vi "start scan.vi"(0 "Experiment name":string, 2 "Scan Number":i32, 5 "Scan":T3 {"Scan setup"."Scan Start" format="%#.9p"; "Scan setup"."Scan End" format="%#.9p"; "Scan setup"."Scan Step Size" format="%#.9p"}, 7 "Network":T5, 12 "BG override":bool, 13 "number BG shots DB":i32, 14 "No of BackGround Shots":i32=2) -> (4 "Scan out":T3 {"Scan setup"."Scan Start" format="%#.9p"; "Scan setup"."Scan End" format="%#.9p"; "Scan setup"."Scan Step Size" format="%#.9p"}, 6 "DoScan":bool, 8 "Network out":T5)   [LabVIEW 2018]
uses:
  MCports.ctl
  Scan Tab Enum.ctl
  scan parameters.ctl
  Shared/MySQL/Preset Query Enum.ctl
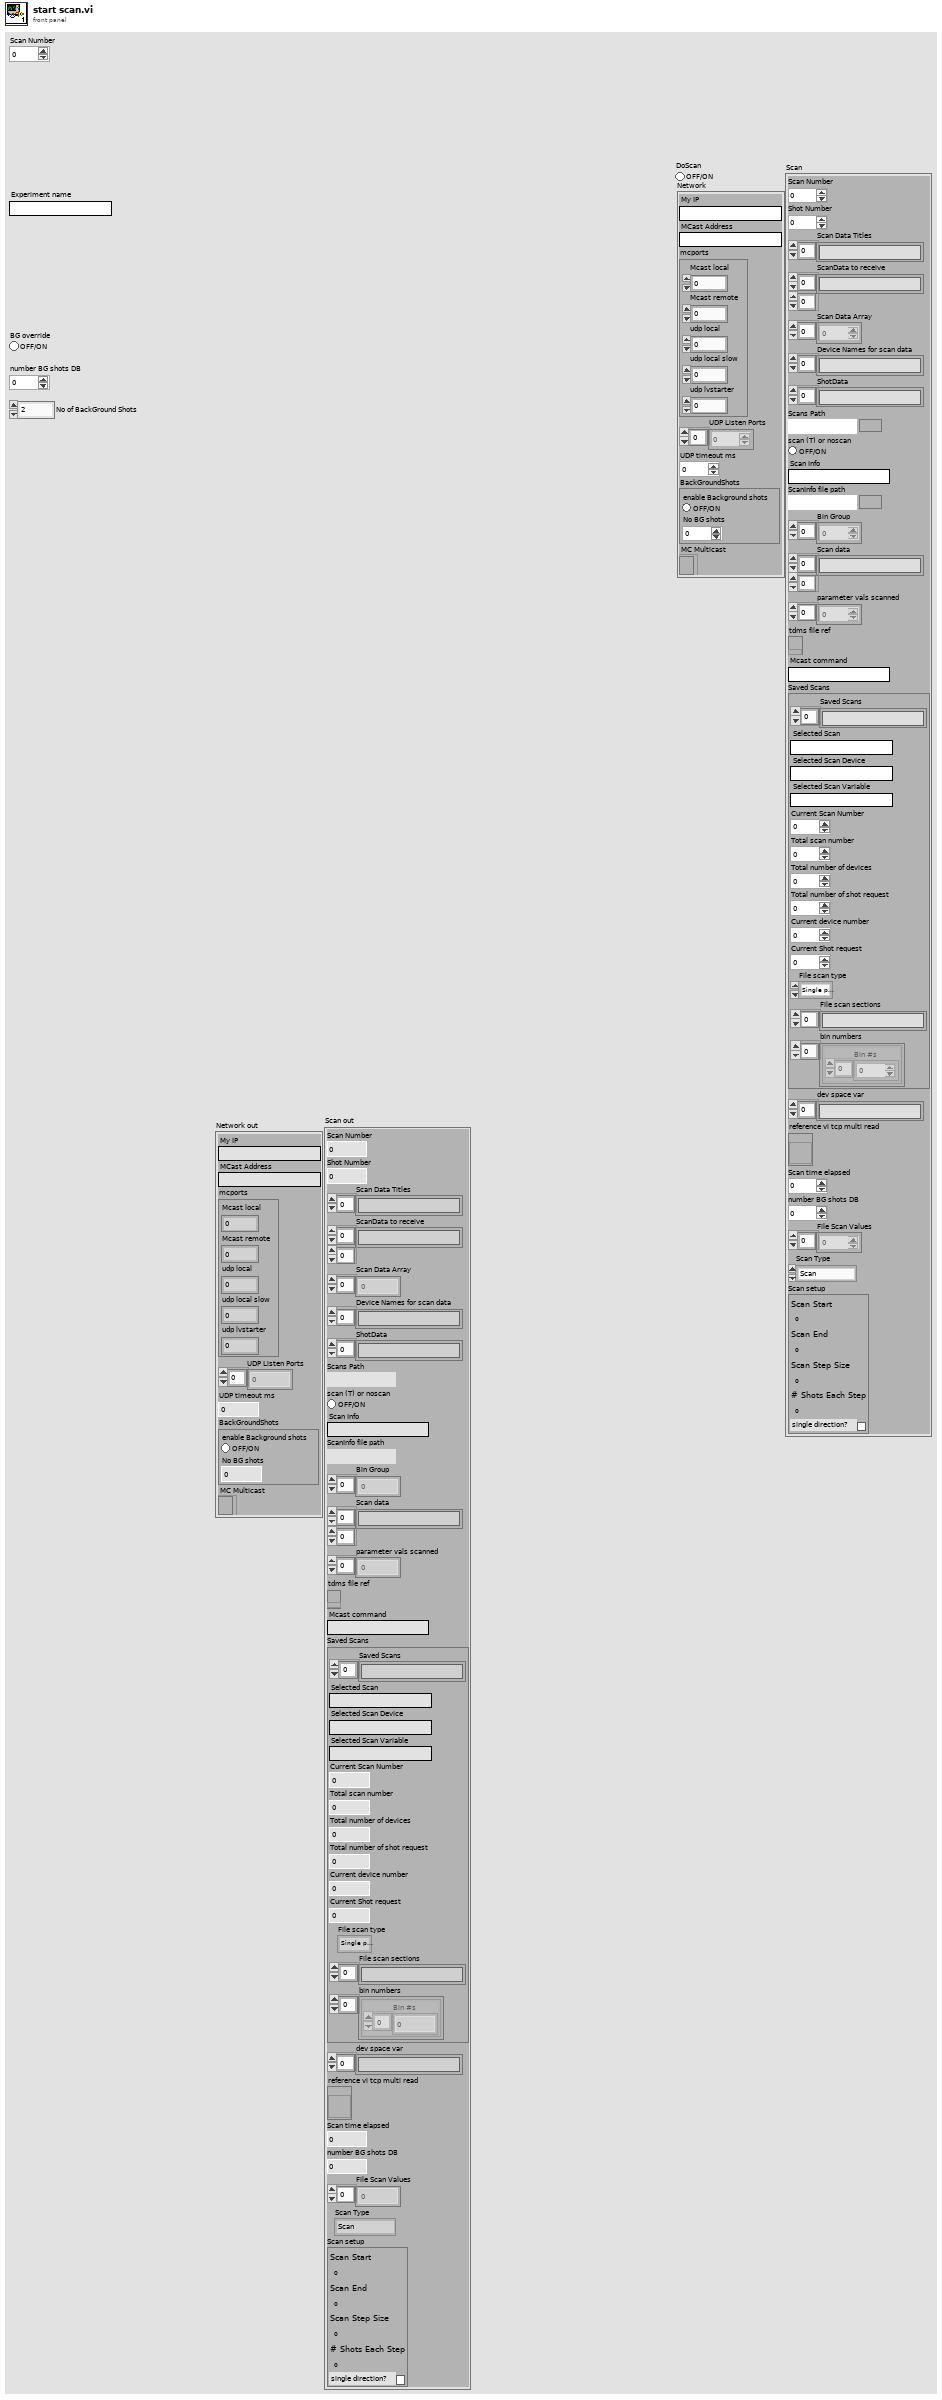
[diagram p1: front panel]
types:
  T1 = typedef "Scan Tab Enum.ctl" = enum32{"Scan", "File Scan", "NoScan", "Saved Scans"}
  T2 = typedef "scan parameters.ctl" = cluster{"Scan Start":dbl, "Scan End":dbl, "Scan Step Size":dbl, "# Shots Each Step":u32, "single direction?":bool}
  T3 = cluster{"Scan Number":i32, "Shot Number":i32, "Scan Data Titles":string[], "ScanData to receive":string[][], "Scan Data Array":dbl[], "Device Names for scan data":string[], "ShotData":string[], "Scans Path":path, "scan (T) or noscan":bool, "Scan Info":string, "ScanInfo file path":path, "Bin Group":i32[], "Scan data":string[][], "parameter vals scanned":dbl[], "tdms file ref":refnum<k34>, "Mcast command":string, "Saved Scans":cluster{"Saved Scans":string[], "Selected Scan":string, "Selected Scan Device":string, "Selected Scan Variable":string, "Current Scan Number":i32, "Total scan number":i32, "Total number of devices":i32, "Total number of shot request":i32, "Current device number":i32, "Current Shot request":i32, "File scan type":enum32{"Single parameter scan", "Multi parameter scan"}, "File scan sections":string[], "bin numbers":cluster{"Bin #s":i32[]}[]}, "dev space var":string[], "reference vi tcp multi read":refnum<vi>, "Scan time elapsed":sgl, "number BG shots DB":i32, "File Scan Values":dbl[], "Scan Type":T1, "Scan setup":T2}
  T4 = typedef "MCports.ctl" = cluster{"Mcast local":u16, "Mcast remote":u16, "udp local":u16, "udp local slow":u16, "udp lvstarter":u16}
  T5 = cluster{"My IP":string, "MCast Address":string, "mcports":T4, "UDP Listen Ports":u16[], "UDP timeout ms":i32, "BackGroundShots":cluster{"enable Background shots":bool, "No BG shots":i32}, "MC Multicast":refnum<k16>}
  T6 = typedef "Preset Query Enum.ctl" = enum16{"Get Locations", "Get all IPs and MACs", "Get classes", "Get expt variables to set at scanstart for particular device", "Get expt devices and variables with start values", "Get expt devices and variables (with data to get)", "Get expt devices with data to get", "Get Expt devices and GUIs", "Get all devices basic properties", "Get Virtual Devices Core Info", "Get Expt names", "Get experiment basic properties", "Get experiment alarm variables", "Get MC Ports", "Get device network comm port", "Get devicetype lvclass path", "Get basic device properties", "Get Init Order", "Get all setable variables of a device", "Get device variable aliases", "Get force values of all settable variables", "Get all variables of a devicetype", "Get all variables of a device", "Get plotter details", "Get Saved Scans", "Get Scan Info", "GetGeneralGUIs", "Get expt for plotter", "Get plotter IDs from expt", "Get all devices", "Get all Virtual Devices", "Get all aliases", "Get variable and device info for Virtual Device", "GetItemLocatorIP", "Get IPs for GUIs", "Get DeviceType from Device", "GetLocalPortRange", "GetDevicePresetVariables", "Get Device Configuration", "GetAllPresetNames", "GetAllConfigurationNames", "GetPresetDeviceNames"}
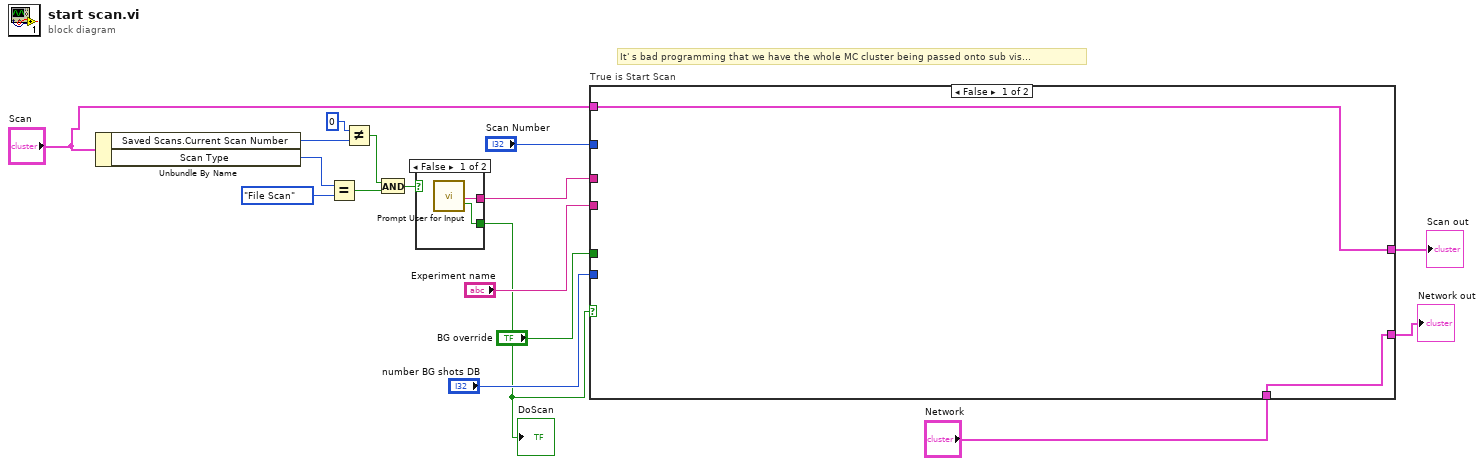
[diagram p0: block diagram]
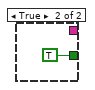
[diagram p2: hidden frame]
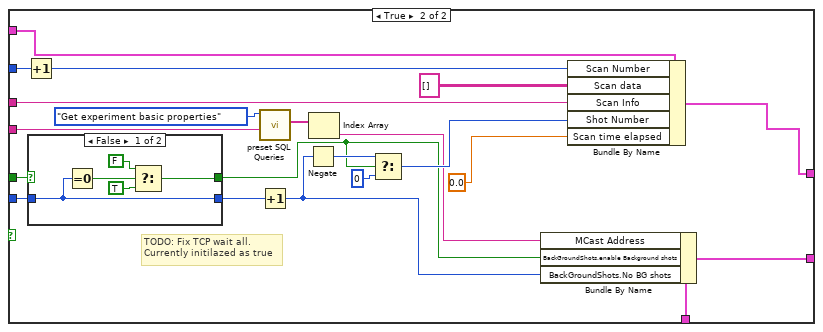
[diagram p3: hidden frame]
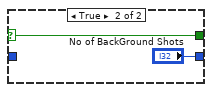
[diagram p4: hidden frame]
diagram:
  # "It' s bad programming that we have the whole MC cluster being passed onto sub vis..."
  n1 = Unbundle By Name("Scan") -> ("Saved Scans.Current Scan Number"=w9:i32, "Scan Type"=w11:T1)
  n2 = Equal?(x=w11, y=Scan_Tab_Enum."File Scan" ("Scan.Scan Type")) -> (x = y?=w6:bool)
  n3 = Not Equal?(x=0, y=w9) -> (x != y?=w7:bool)
  n4 = And(x=w7, y=w6) -> (x .and. y?=w5:bool)
  n5 = case shown="False" w5 {
    tunnel: [w19 _] -> w13
    tunnel: [w18 TRUE ("OK")] -> w12
    frame False {
      n6 = call "Prompt User for Input"() -> ("Scan information"=w19:string, "OK"=w18:bool)  [unwired: 17 in, 1 out]
    }
    frame True {
    }
  }
  "DoScan" <- w12
  n7 = case "True is Start Scan" shown="False" w12 {
    tunnel: "Scan" -> [w21 w24]
    tunnel: "Scan Number" -> [_ w43]
    tunnel: "Experiment name" -> [_ w39]
    tunnel: "number BG shots DB" -> [_ w32]
    tunnel: "BG override" -> [_ w31]
    tunnel: w13 -> [_ w30]
    tunnel: [w22 w26] -> w4
    tunnel: "Network" -> [w22 w25]
    tunnel: [w21 w23] -> w1
    frame False {
    }
    frame True {
      # "TODO: Fix TCP wait all. \nCurrently initilazed as true"
      n8 = Increment(x=w43) -> (x+1=w42:i32)
      n9 = case shown="False" w31 {
        selector: w31 -> [_ w49]
        tunnel: [w45 "No of BackGround Shots"] -> w33
        tunnel: [w44 w49] -> w28
        tunnel: w32 -> [w45 _]
        frame False {
          n10 = Equal To 0?(x=w45) -> (x = 0?=w48:bool)
          n11 = Select(t=FALSE ("BG override"), s=w48, f=TRUE) -> (s? t:f=w44:bool)
        }
        frame True {
        }
      }
      n12 = call "preset SQL Queries.vi"("Expt name / MCIP/ Variable/Preset Name"=w39, "Preset Query"=Preset_Query_Enum."Get experiment basic properties") -> ("1st column 1st data"=w38:string[])  [unwired: 7 in, 2 out]
      n13 = Increment(x=w33) -> (x+1=w27:i32)
      n14 = Negate(x=w27) -> (-x=w34:i32)
      n15 = Index Array(array=w38) -> (element=w29:string)  [unwired: 1 in]
      n16 = Select(t=w34, s=w28, f=0 ("Shot Number")) -> (s? t:f=w37:i32)
      n17 = Bundle By Name(cluster=w25, "MCast Address"=w29, "BackGroundShots.enable Background shots"=w28, "BackGroundShots.No BG shots"=w27) -> (w26:T5)
      n18 = Bundle By Name(cluster=w24, "Scan Number"=w42, "Scan data"=string[][] [], "Scan Info"=w30, "Shot Number"=w37, "Scan time elapsed"=sgl 0.0 ("Scan.Scan time elapsed")) -> (w23:T3)
    }
  }
  "Network out" <- w4
  "Scan out" <- w1
